vi "配置参数转换为字符串.vi"(1 "配置参数":T1 {"标准最低转速" format="%0.1f rpm"; "标准最高转速" format="%0.1f rpm"; "积分调节时间" format="%#.1f"; "比例调节增益" format="%#.1g%%"; "速差曲线点4" format="%#.1g%%"; "速差曲线点2" format="%#.1g%%"; "速差曲线点3" format="%#.1g%%"; "速差曲线点1" format="%#.1g%%"; "速差曲线点4 反馈" format="%#.1g%%"; "速差曲线点2 反馈" format="%#.1g%%"; "速差曲线点3 反馈" format="%#.1g%%"; "速差曲线点1 反馈" format="%#.1g%%"; "最低转速" format="%#.1f"; "最高转速" format="%#.1f"; "测速盘齿数" format="%#.0f"; "DEH内置参数值" format="%.1f %"}) -> (0 "String":string)   [LabVIEW 2013]
panel:
  # "调节参数"
  # "阀门输出"
  # "转速反馈"
  # "速差曲线点"
  # "反馈"
  # "DEH"
  # "LVDT 1"
  # "LVDT 2"
  # "DEH"
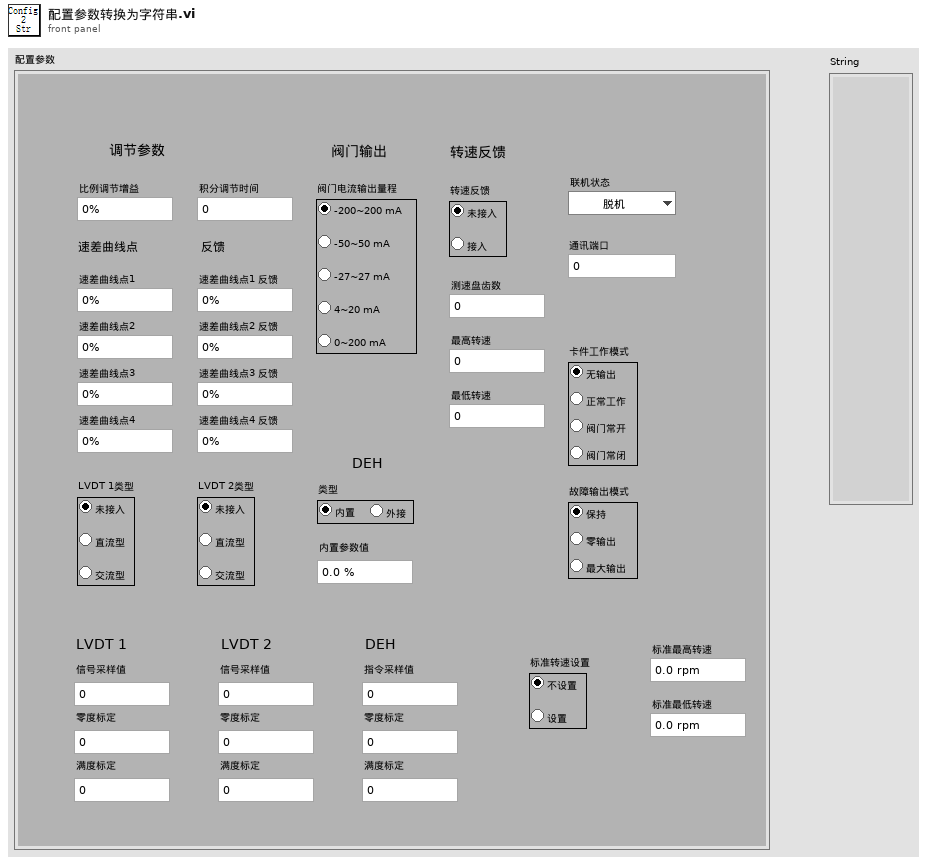
[diagram p1: front panel]
types:
  T1 = cluster{"卡件工作模式":enum32{"未接入", "直流型", "交流型", "交流型 2"}, "转速反馈":enum32{"未接入", "直流型"}, "故障输出模式":enum32{"未接入", "直流型", "交流型"}, "DEH类型":enum32{"内置", "外接"}, "LVDT 2类型":enum32{"未接入", "直流", "交流"}, "LVDT 1类型":enum32{"未接入", "直流", "交流"}, "阀门电流输出量程":enum32{"-200~200 mA", "-50~50 mA", "-27~27 mA", "4~20 mA", "0~200 mA"}, "DEH内置参数值":dbl, "测速盘齿数":dbl, "最高转速":dbl, "最低转速":dbl, "速差曲线点1 反馈":dbl, "速差曲线点3 反馈":dbl, "速差曲线点2 反馈":dbl, "速差曲线点4 反馈":dbl, "速差曲线点1":dbl, "速差曲线点3":dbl, "速差曲线点2":dbl, "速差曲线点4":dbl, "比例调节增益":dbl, "积分调节时间":dbl, "通讯端口":dbl, "联机状态":enum16{"脱机", "联机"}, "DEH零度标定":dbl, "DEH满度标定":dbl, "DEH指令采样值":dbl, "LVDT 2零度标定":dbl, "LVDT 2满度标定":dbl, "LVDT 2信号采样值":dbl, "LVDT 1零度标定":dbl, "LVDT 1满度标定":dbl, "LVDT1 信号采样值":dbl, "标准最高转速":dbl, "标准最低转速":dbl, "标准转速设置":enum32{"未接入", "直流型"}}
  T2 = enum32{"-200~200 mA", "-50~50 mA", "-27~27 mA", "4~20 mA", "0~200 mA"}
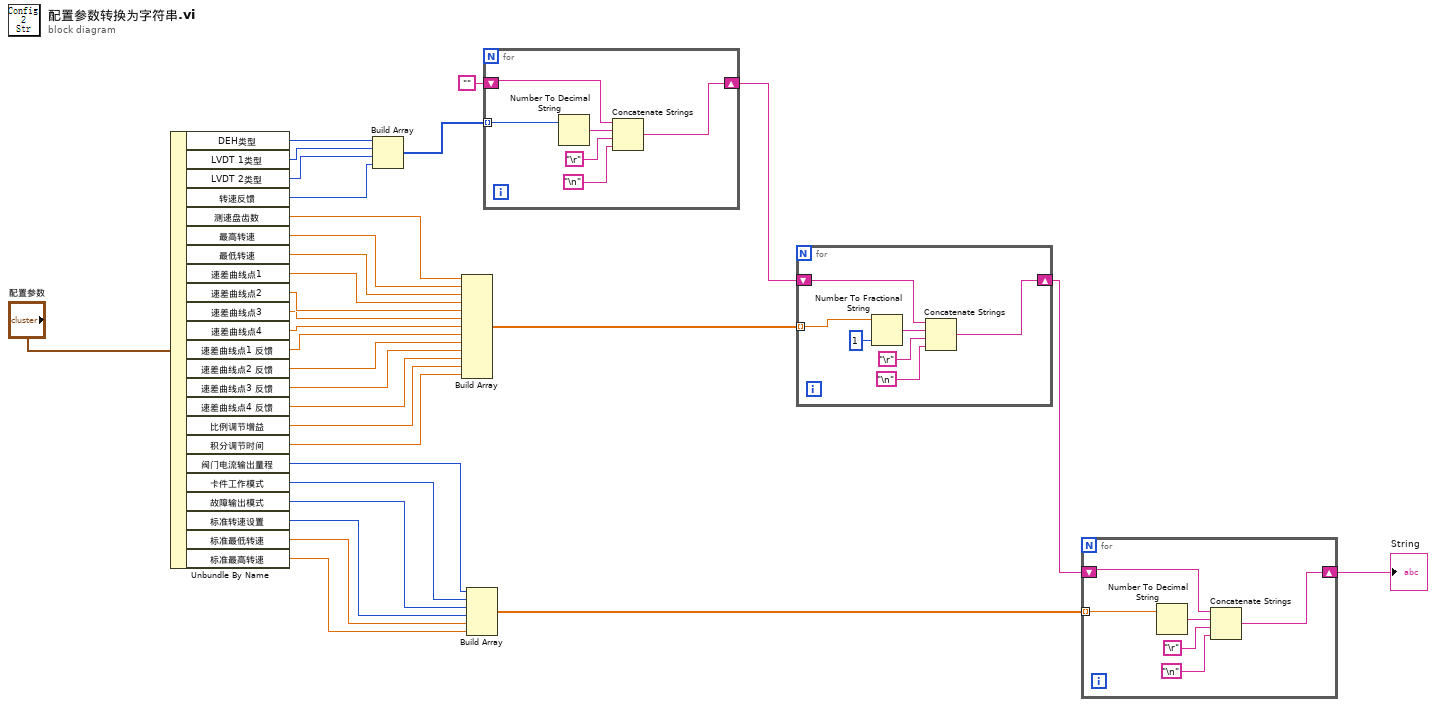
[diagram p0: block diagram]
diagram:
  n1 = Unbundle By Name("配置参数") -> ("DEH类型"=w11:enum32{"内置", "外接"}, "LVDT 1类型"=w10:enum32{"未接入", "直流", "交流"}, "LVDT 2类型"=w9:enum32{"未接入", "直流", "交流"}, "转速反馈"=w8:enum32{"未接入", "直流型"}, "测速盘齿数"=w31:dbl, "最高转速"=w30:dbl, "最低转速"=w29:dbl, "速差曲线点1"=w28:dbl, "速差曲线点2"=w27:dbl, "速差曲线点3"=w26:dbl, "速差曲线点4"=w25:dbl, "速差曲线点1 反馈"=w24:dbl, "速差曲线点2 反馈"=w23:dbl, "速差曲线点3 反馈"=w22:dbl, "速差曲线点4 反馈"=w21:dbl, "比例调节增益"=w20:dbl, "积分调节时间"=w19:dbl, "阀门电流输出量程"=w17:T2, "卡件工作模式"=w16:enum32{"未接入", "直流型", "交流型", "交流型 2"}, "故障输出模式"=w15:enum32{"未接入", "直流型", "交流型"}, "标准转速设置"=w3:enum32{"未接入", "直流型"}, "标准最低转速"=w2:dbl, "标准最高转速"=w1:dbl)
  n2 = Build Array(w11, w10, w9, w8) -> (w7:u32[])
  n3 = Build Array(w31, w30, w29, w28, w27, w26, w25, w24, w23, w22, w21, w20, w19) -> (w18:dbl[])
  n4 = Build Array(w17, w16, w15, w3, w2, w1) -> (w14:dbl[])
  n5 = for {
    tunnel: w7 -> [w32] mode=indexing
    shift-right: [w34] -> w5
    shift-left: "" -> [w33]
    n6 = Number To Decimal String(number=w32) -> (decimal integer string=w37:string)  [unwired: 1 in]
    n7 = Concatenate Strings(w33, w37, "\r", "\n") -> (w34:string)
  }
  n8 = for {
    tunnel: w18 -> [w38] mode=indexing
    shift-right: [w40] -> w13
    shift-left: w5 -> [w39]
    n9 = Number To Fractional String(number=w38, precision (6)=i16 1) -> (F-format string=w43:string)  [unwired: 2 in]
    n10 = Concatenate Strings(w39, w43, "\r", "\n") -> (w40:string)
  }
  n11 = for {
    tunnel: w14 -> [w45] mode=indexing
    shift-right: [w47] -> w12
    shift-left: w13 -> [w46]
    n12 = Number To Decimal String(number=w45) -> (decimal integer string=w50:string)  [unwired: 1 in]
    n13 = Concatenate Strings(w46, w50, "\r", "\n") -> (w47:string)
  }
  "String" <- w12
